vi "Thread Page.vi"(8 "error in (no error)":errorcluster, 11 "Node Ptr":T1 format="%.0x") -> (0 "error out":errorcluster)   [LabVIEW 2019, in "DSF System Explorer.lvlib"]
uses:
  DSF System Explorer.lvlib
  <vilib>/NI VeriStand/Custom Device API/Custom Device API.lvlib
  Shared/DSF Shared.lvlib
  DSF Core.lvlibp/Classes/Component User Interface/UI Type.ctl
  <vilib>/NI VeriStand/Custom Device API/Custom Device Item Ref.ctl
panel:
  in  "Tab Control":enum32{"Settings"}(tab)
  in  "Processor":i32
  in  "Priority Offset":i16
  in  "Header":cluster{"Section Name":string}={"Section Name"="Thread"}
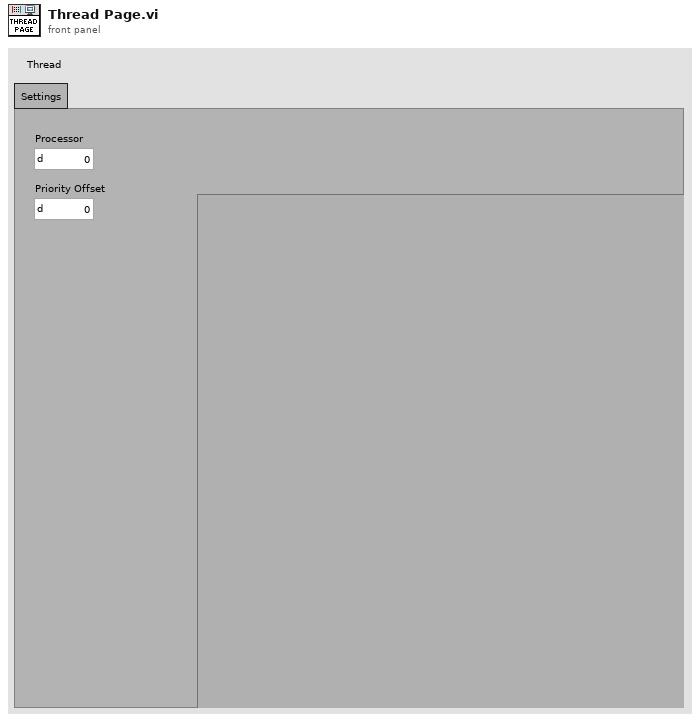
[diagram p1: front panel]
types:
  T1 = typedef "Custom Device API.lvlib/Custom Device Item Ref.ctl" = u64
  T2 = typedef "DSF Core.lvlibp/Component User Interfaces.lvclass/UI Type.ctl" = enum16{"Plugin", "Thread", "Rx Group", "Tx Group", "Rx Transfer", "Tx Transfer", "Rx Channel", "Tx Channel"}
  T3 = typedef "DSF Core.lvlibp/Thread Configuration.lvclass/Core Thread Configuration.ctl" = cluster{"processor":i32, "priority offset":i16}
  T4 = typedef "DSF Core.lvlibp/User Interface Handler.lvclass/User Interface Ref.ctl" = refnum<vi>
  T5 = typedef "DSF Core.lvlibp/DSF Settings Info.ctl" = cluster{"component":string, "values":cluster{"key":string, "value":string}[]}
  T6 = typedef "Custom Device API.lvlib/Custom Device Commands.ctl" = enum16{"Default", "Item renamed", "Shutdown", "Dynamic button pressed"}
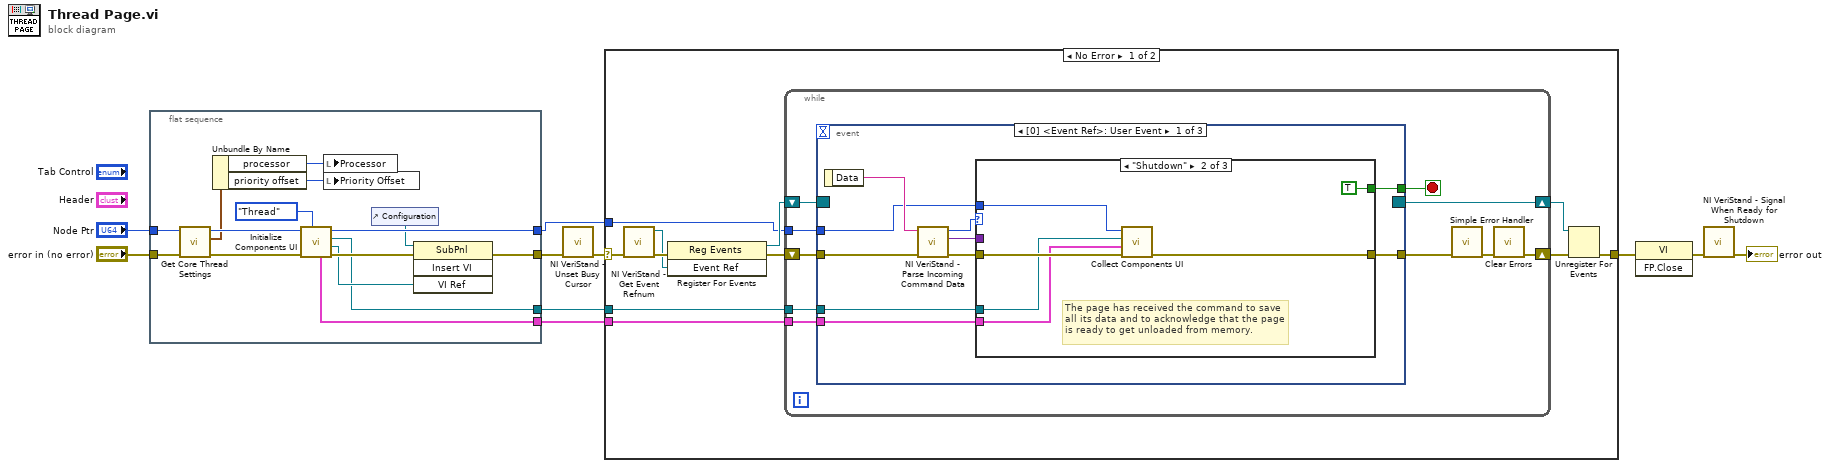
[diagram p0: block diagram]
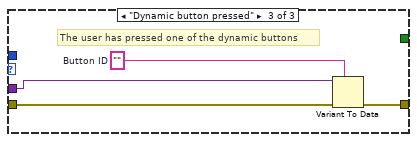
[diagram p3: hidden frame]
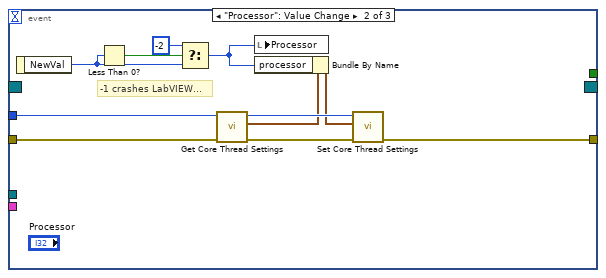
[diagram p4: hidden frame]
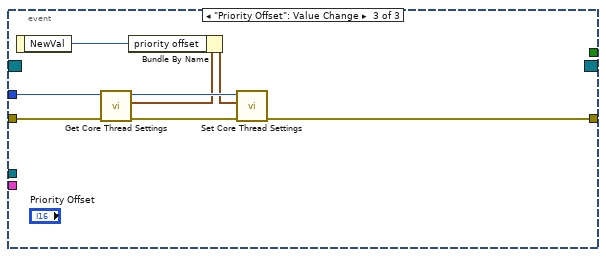
[diagram p5: hidden frame]
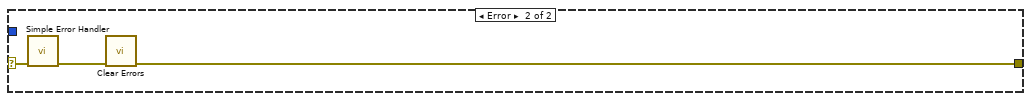
[diagram p6: hidden frame]
diagram:
  n1 = flat-sequence "Initialization code" {
    tunnel: "error in (no error)" -> [w25]
    tunnel: "Node Ptr" -> [w24]
    tunnel: [w18] -> w4
    tunnel: [w14] -> w3
    tunnel: [w13] -> w2
    tunnel: [w11] -> w1
    frame #0 {
      n2 = call "Get Core Thread Settings.vi"("error in (no error)"=w25, "Item Ref in"=w24) -> ("error out"=w20:errorcluster, "thread configuration"=w17:T3, "Item Ref out"=w19:T1)  [unwired: 7 in]
      n3 = Unbundle By Name(w17) -> ("processor"=w23:i32, "priority offset"=w22:i16)
      n4 = call "Initialize Components UI.vi"("user interface type"=UI_Type."Thread", "error in (no error)"=w20, "Item Ref in"=w19) -> ("error out"=w16:errorcluster, "active vi"=w15:T4, "User Interface Handler"=w14:refnum<class "User Interface Handler.lvclass">, "Item Ref out"=w18:T1, "component settings"=w11:T5[])  [unwired: 4 in]
      n5 = local write "Processor"(w23) -> ()
      n6 = local write "Priority Offset"(w22) -> ()
      n7 = control-ref of="Configuration"() -> (w12:refnum<vi>)
      n8 = invoke class="SubPnl" method="Insert VI"(reference=w12, error in=w16, "VI Ref"=w15) -> (error out=w13:errorcluster)  [unwired: 1 in, 3 out]
    }
  }
  n9 = call <vilib>:"NI VeriStand - Unset Busy Cursor.vi"("error in (no error)"=w2) -> ("error out"=w6:errorcluster)  [unwired: 10 out]
  n10 = case shown="No Error" w6 {
    selector: w6 -> [w28 w89]
    tunnel: [w33 w87] -> w10
    tunnel: w4 -> [w29 _]
    tunnel: w3 -> [w27 _]
    tunnel: w1 -> [w26 _]
    frame No Error {
      n11 = call <vilib>:"NI VeriStand - Get Event Refnum.vi"("error in (no error)"=w28) -> ("error out"=w36:errorcluster, "Event Ref"=w32:refnum<user-event>)  [unwired: 9 out]
      n12 = register-events(error in=w36, w32) -> (reference out=w30:refnum<event-registration>, error out=w31:errorcluster)  [unwired: 1 in]
      n13 = while {
        tunnel: w29 -> [w42]
        shift-right: [w39] -> w34
        shift-left: w31 -> [w45]
        shift-right: [w46] -> w35
        shift-left: w30 -> [w44]
        tunnel: w27 -> [w38]
        tunnel: w26 -> [w37]
        stop <- w43 stop-if-true
        n14 = event shown="[0] <Event Ref>: User Event" {
          selector: w44 -> [_ _ _]
          dyn-events: [_ _ _] -> w46
          timeout: _ -> [_ _ _]
          tunnel: w45 -> [w56 w78 w86]
          tunnel: [w52 _ _] -> w43
          tunnel: [w51 w72 w79] -> w41
          tunnel: w42 -> [w50 w77 w85]
          tunnel: w38 -> [w48 _ _]
          tunnel: w37 -> [w47 _ _]
          event User Event {
            n15 = event-data() -> ("Data"=w55:string)  [unwired: 1 out]
            n16 = call <vilib>:"NI VeriStand - Parse Incoming Command Data.vi"("error in (no error)"=w56, "Incoming data"=w55) -> ("error out"=w54:errorcluster, "Outgoing data"=w49:variant, "Action"=w53:T6)  [unwired: 7 out]
            n17 = case shown="\"Shutdown\"" w53 {
              tunnel: w54 -> [w57 w62 w67]
              tunnel: [_ TRUE _] -> w52
              tunnel: [w57 w61 w64] -> w51
              tunnel: w50 -> [_ w60 _]
              tunnel: w49 -> [_ _ w66]
              tunnel: w48 -> [_ w59 _]
              tunnel: w47 -> [_ w58 _]
              frame "Default", Default {
              }
              frame "Shutdown" {
                # "The page has received the command to save all its data and to acknowledge that the page is ready to get unloaded from memory."
                n18 = call "Collect Components UI.vi"("error in (no error)"=w62, "current component settings"=w58, "User Interface Handler"=w59, "Item Ref in"=w60) -> ("error out"=w61:errorcluster)  [unwired: 6 in, 1 out]
              }
              frame "Dynamic button pressed" {
                w65 = ""  # Button ID
                # "The user has pressed one of the dynamic buttons"
                n19 = Variant To Data(error in=w67, type=w65, Variant=w66) -> (error out=w64:errorcluster)  [unwired: 1 out]
              }
            }
          }
          event "Processor": Value Change {
            # "-1 crashes LabVIEW..."
            n20 = event-data() -> ("NewVal"=w70:i32)  [unwired: 1 out]
            n21 = Less Than 0?(x=w70) -> (x < 0?=w71:bool)
            n22 = Select(t=-2, s=w71, f=w70) -> (s? t:f=w69:i32)
            n23 = call "Get Core Thread Settings.vi"("error in (no error)"=w78, "Item Ref in"=w77) -> ("error out"=w73:errorcluster, "thread configuration"=w75:T3, "Item Ref out"=w76:T1)  [unwired: 7 in]
            n24 = local write "Processor"(w69) -> ()
            n25 = Bundle By Name(cluster=w75, "processor"=w69) -> (w74:T3)
            n26 = call "Set Core Thread Settings.vi"("error in (no error)"=w73, "thread configuration"=w74, "Item Ref in"=w76) -> ("error out"=w72:errorcluster)  [unwired: 7 in, 1 out]
          }
          event "Priority Offset": Value Change {
            n27 = event-data() -> ("NewVal"=w84:i16)  [unwired: 1 out]
            n28 = call "Get Core Thread Settings.vi"("error in (no error)"=w86, "Item Ref in"=w85) -> ("error out"=w80:errorcluster, "thread configuration"=w82:T3, "Item Ref out"=w83:T1)  [unwired: 7 in]
            n29 = Bundle By Name(cluster=w82, "priority offset"=w84) -> (w81:T3)
            n30 = call "Set Core Thread Settings.vi"("error in (no error)"=w80, "thread configuration"=w81, "Item Ref in"=w83) -> ("error out"=w79:errorcluster)  [unwired: 7 in, 1 out]
          }
        }
        n31 = call <vilib>:"Simple Error Handler.vi"("error in (no error)"=w41) -> ("error out"=w40:errorcluster)  [unwired: 1 in, 7 out]
        n32 = call <vilib>:"Clear Errors.vi"("error in (no error)"=w40) -> ("error out"=w39:errorcluster)  [unwired: 1 in, 5 out]
      }
      n33 = Unregister For Events(event registration refnum=w35, error in=w34) -> (error out=w33:errorcluster)
    }
    frame Error {
      n34 = call <vilib>:"Simple Error Handler.vi"("error in (no error)"=w89) -> ("error out"=w88:errorcluster)  [unwired: 1 in, 7 out]
      n35 = call <vilib>:"Clear Errors.vi"("error in (no error)"=w88) -> ("error out"=w87:errorcluster)  [unwired: 1 in, 5 out]
    }
  }
  n36 = invoke class="VI" method="FP.Close"(error in=w10) -> (error out=w9:errorcluster)  [unwired: 2 in, 2 out]
  n37 = call <vilib>:"NI VeriStand - Signal When Ready for Shutdown.vi"("error in (no error)"=w9) -> ("error out"=→"error out":errorcluster)  [unwired: 10 out]
